vi "Initialize Motor Communication.vi"(8 "error in (no error)":errorcluster, 11 "motor name (unnamed)":string) -> (0 "error out":errorcluster, 3 "motor communication out":refnum<class "NI_Robotics_Motor Communication.lvclass">)   [LabVIEW 2017, in "NI_Robotics_Motor Communication.lvclass"]
doc: "Begins a communication session for the motor that controls the wheel you specify."
uses:
  <vilib>/robotics/Actuation/Motor Communication/NI_Robotics_Motor Communication.lvclass
  <vilib>/robotics/Actuation/Motor Communication Ref/NI_Robotics_Motor Communication Ref.lvclass
  c:/Program Files (x86)/National Instruments/LabVIEW 2017/vi.lib/robotics/Actuation/Motor Communication/NI_Robotics_Motor Communication.lvclass
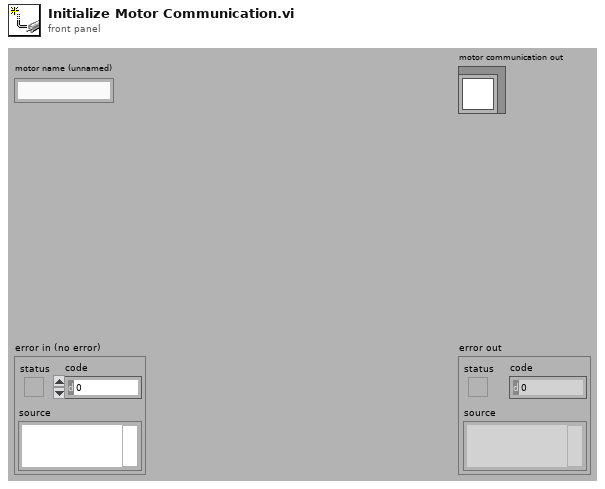
[diagram p1: front panel]
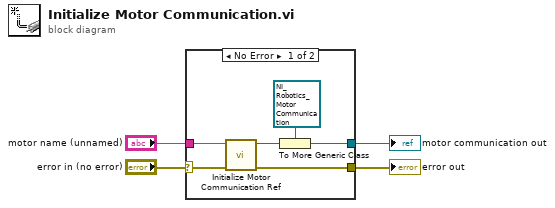
[diagram p0: block diagram]
diagram:
  n1 = case shown="No Error" "error in (no error)" {
    selector: "error in (no error)" -> [w10 w11]
    tunnel: [w9 w11] -> w3
    tunnel: "motor name (unnamed)" -> [w5 _]
    tunnel: [w7 _] -> w1
    frame No Error {
      n2 = call <vilib>:"Initialize Motor Communication Ref.vi"("error in (no error)"=w10, "motor name (unnamed)"=w5) -> ("error out"=w9:errorcluster, "motor communication ref out"=w8:refnum<class "NI_Robotics_Motor Communication Ref.lvclass">)  [unwired: 8 in]
      n3 = To More Generic Class(target class=refnum<class "NI_Robotics_Motor Communication.lvclass"> refnum ("NI_Robotics_Motor Communication.lvclass"), reference=w8) -> (generic class reference=w7:refnum<class "NI_Robotics_Motor Communication.lvclass">)
    }
    frame Error {
    }
  }
  "error out" <- w3
  "motor communication out" <- w1
